vi "SetMeasureOverlapBuffer.vi"(7 "SMU":T2, 8 "Error In":errorcluster, 9 "Buffer":string="(rbuffer)", 10 "Measure Function":T1, 11 "Keithley 2602 In":refnum<visa-resource-name>) -> (0 "Error Out":errorcluster, 3 "Keithley 2602 Out":refnum<visa-resource-name>)   [LabVIEW 2012, in "Keithley-2602.lvlib"]
uses:
  Keithley-2602.lvlib
  Controls/SMU.ctl
  Controls/MeasureFunction.ctl
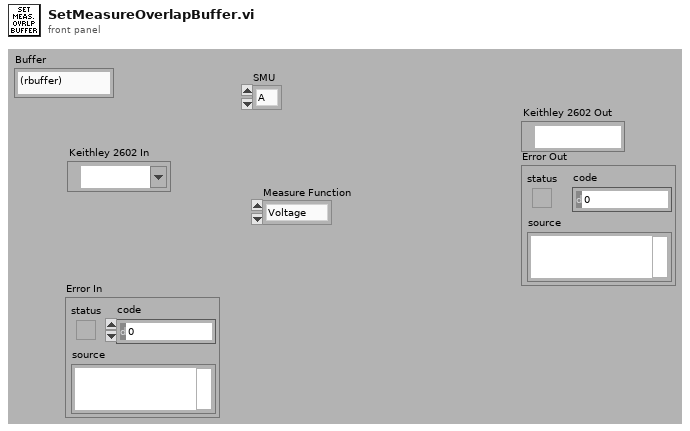
[diagram p1: front panel]
types:
  T1 = typedef "Keithley-2602.lvlib/MeasureFunction.ctl" = enum16{"Voltage", "Current", "Resistance", "Power"}
  T2 = typedef "Keithley-2602.lvlib/SMU.ctl" = enum16{"A", "B"}
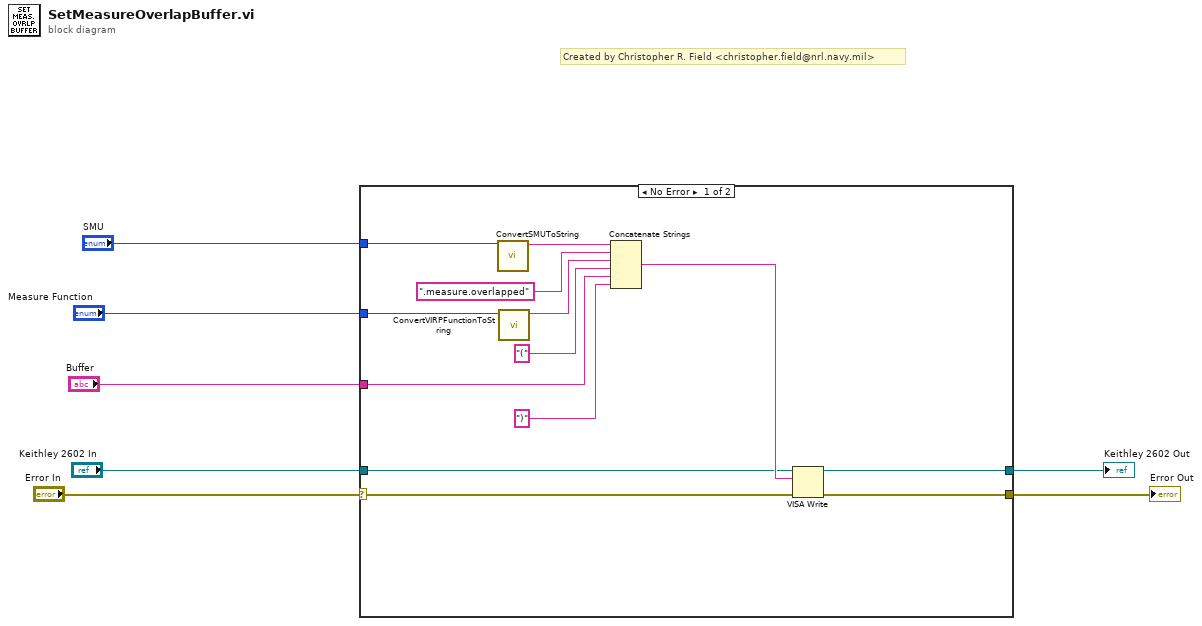
[diagram p0: block diagram]
diagram:
  # "Created by Christopher R. Field <christopher.field@nrl.navy.mil>"
  n1 = case shown="No Error" "Error In" {
    selector: "Error In" -> [w8 w21]
    tunnel: "Keithley 2602 In" -> [w18 w22]
    tunnel: [w17 w22] -> w6
    tunnel: [w16 w21] -> w5
    tunnel: "Buffer" -> [w12 _]
    tunnel: "Measure Function" -> [w10 _]
    tunnel: "SMU" -> [w9 _]
    frame No Error {
      n2 = call "ConvertSMUToString.vi"("SMU"=w9) -> ("Channel"=w15:string)  [unwired: 10 in]
      n3 = call "ConvertVIRPFunctionToString.vi"("Function"=w10) -> ("Function"=w14:string)  [unwired: 10 in]
      n4 = Concatenate Strings(w15, ".measure.overlapped", w14, "(" ("string"), w12, ")" ("string")) -> (w19:string)
      n5 = VISA Write(VISA resource name=w18, write buffer=w19, error in (no error)=w8) -> (VISA resource name out=w17:refnum<visa-resource-name>, error out=w16:errorcluster)  [unwired: 1 out]
    }
    frame Error {
    }
  }
  "Keithley 2602 Out" <- w6
  "Error Out" <- w5
